vi "GetType.vi"(8 "error in (no error)":errorcluster, 11 "Add Data without TS Msg":refnum<class "Add Data without TS Msg.lvclass">) -> (0 "error out":errorcluster, 2 "Data Sample":variant, 3 "Add Data without TS Msg":refnum<class "Add Data without TS Msg.lvclass">)   [LabVIEW 2018, in "BNT_XtGraph.lvlib" / "Add Data without TS Msg.lvclass"]
uses:
  Add Data without TS Msg.lvclass
  Add Data without TS Msg.lvclass/Add Data without TS Msg.ctl
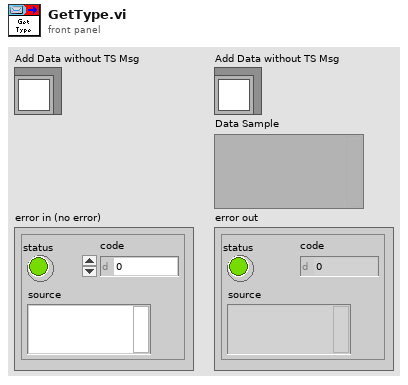
[diagram p1: front panel]
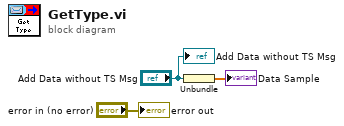
[diagram p0: block diagram]
diagram:
  n1 = Unbundle("Add Data without TS Msg") -> (→"Data Sample":dbl[])
  "error out" <- "error in (no error)"
  "Add Data without TS Msg" <- "Add Data without TS Msg"
